vi "Stream Data I64x2.vi"(0 "i in":fxp<+/-,64,1>, 5 "q in":fxp<+/-,64,1>, 7 "config":T3, 9 "input valid":bool) -> (6 "status":T2)   [LabVIEW 2017, in "Lock-In Amplifier Example FPGA.lvlib"]
uses:
  Lock-In Amplifier Example FPGA.lvlib
  <instrlib>/_niInstr/Streaming/v1/Common/Stream State.ctl
  <vilib>/rvi/interface/RandomDataEmulation/niFpgaRandomDataHandleErrors.vi
  <vilib>/rvi/DataTransferAndStorage/Container/XNode/niFpgaContainer.xnode
  <vilib>/rvi/interface/RandomDataEmulation/nirviRandomDataFpgaReadWriteTemplate.vi
  <instrlib>/_niInstr/Streaming/v1/FPGA/niInstr Streaming v1 FPGA.lvlib
  <instrlib>/_niInstr/Streaming/v1/Common/niInstr Streaming v1 Common.lvlib
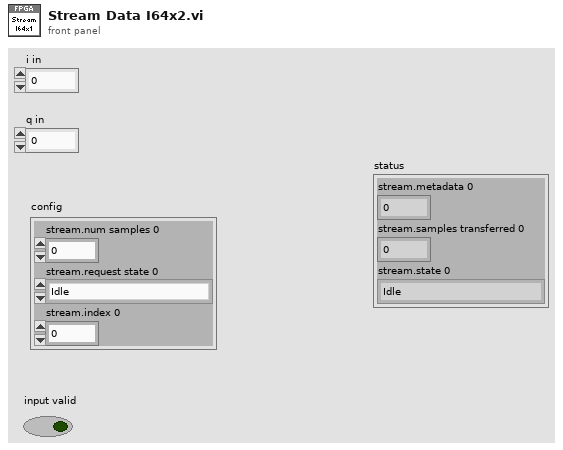
[diagram p1: front panel]
types:
  T1 = typedef "niInstr Streaming v1 Common.lvlib/Stream State.ctl" = enum8{"Idle", "Finite Transfer", "Continuous", "Done", "Error", "Not Ready", "Cancel"}
  T2 = cluster{"stream.metadata 0":u64, "stream.samples transferred 0":u64, "stream.state 0":T1}
  T3 = cluster{"stream.num samples 0":u64, "stream.request state 0":T1, "stream.index 0":i16}
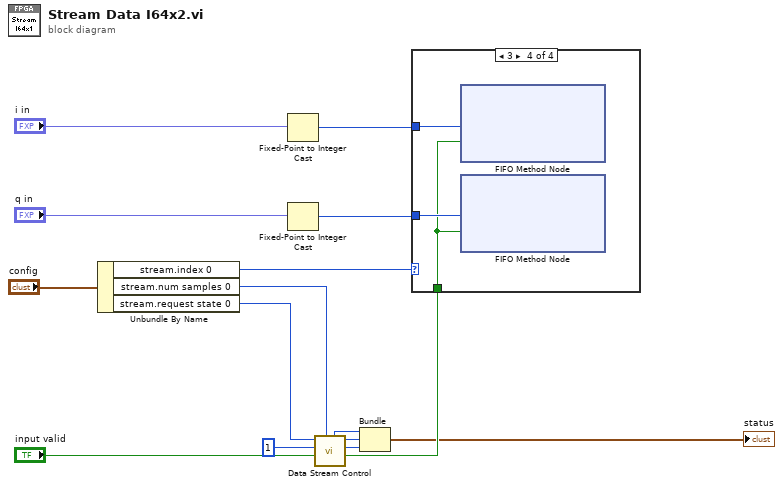
[diagram p0: block diagram]
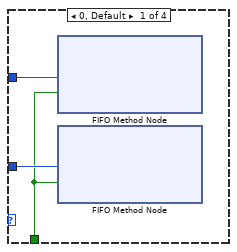
[diagram p2: hidden frame]
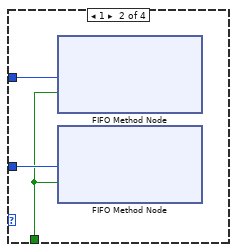
[diagram p3: hidden frame]
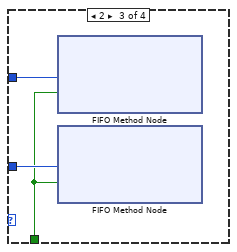
[diagram p4: hidden frame]
diagram:
  n1 = Unbundle By Name("config") -> ("stream.index 0"=w1:i16, "stream.num samples 0"=w7:u64, "stream.request state 0"=w6:T1)
  n2 = Fixed-Point to Integer Cast(1:"i in") -> (0:w12:i64)
  n3 = Fixed-Point to Integer Cast(1:"q in") -> (0:w10:i64)
  n4 = call <instrlib>:"Data Stream Control.vi"("stream.num samples 0"=w7, "data valid"="input valid", "element count"=u16 1, "stream.request state 0"=w6) -> ("send data"=w9:bool, "stream.state 0"=w3:T1, "stream.samples transferred 0"=w4:u64, "stream.metadata 0"=w5:u64)  [unwired: 3 in, 1 out]
  n5 = Bundle("stream.metadata 0"=w5, "stream.samples transferred 0"=w4, "stream.state 0"=w3) -> (→"status":T2)  [unwired: 1 in]
  n6 = case shown="3" w1 {
    tunnel: w12 -> [w18 w21 w24 w27]
    tunnel: w10 -> [w17 w20 w23 w26]
    tunnel: w9 -> [w16 w19 w22 w25]
    frame 0, Default {
      n7 = xnode ("FIFO Method Node")("Element"=w18, "Input Valid"=w16) -> ()  [unwired: 1 in, 2 out]
      n8 = xnode ("FIFO Method Node")("Element"=w17, "Input Valid"=w16) -> ()  [unwired: 1 in, 2 out]
    }
    frame 1 {
      n9 = xnode ("FIFO Method Node")("Element"=w21, "Input Valid"=w19) -> ()  [unwired: 1 in, 2 out]
      n10 = xnode ("FIFO Method Node")("Element"=w20, "Input Valid"=w19) -> ()  [unwired: 1 in, 2 out]
    }
    frame 2 {
      n11 = xnode ("FIFO Method Node")("Element"=w24, "Input Valid"=w22) -> ()  [unwired: 1 in, 2 out]
      n12 = xnode ("FIFO Method Node")("Element"=w23, "Input Valid"=w22) -> ()  [unwired: 1 in, 2 out]
    }
    frame 3 {
      n13 = xnode ("FIFO Method Node")("Element"=w27, "Input Valid"=w25) -> ()  [unwired: 1 in, 2 out]
      n14 = xnode ("FIFO Method Node")("Element"=w26, "Input Valid"=w25) -> ()  [unwired: 1 in, 2 out]
    }
  }
